vi "Get Size of Data from TD - Digital Data (Ramp 256 Samples) - Returns Correct Size.vi"() -> ()   [LabVIEW 2017, in "Composition.Tests.lvlib"]
uses:
  Composition.Tests.lvlib
  <vilib>/Waveform/DWDTOps.llb/Digital Pattern Generator (Ramp).vi
  <vilib>/addons/_JKI Toolkits/Caraya/classes/Assert/Assert Equal Value_Variant.vi
  Composition/Composition.lvlib
  <vilib>/addons/_JKI Toolkits/Caraya/classes/Assert/Assert.lvclass
  <vilib>/addons/_JKI Toolkits/Caraya/classes/Test/Test.lvclass
panel:
  out "error out":errorcluster
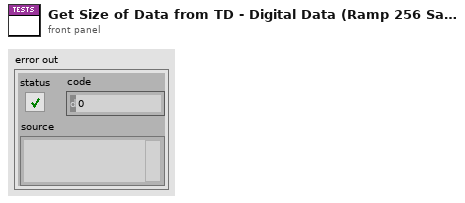
[diagram p1: front panel]
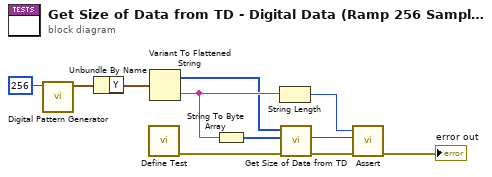
[diagram p0: block diagram]
diagram:
  n1 = call-poly <vilib>:"Digital Pattern Generator.vi"("number of samples"=u32 256) -> ("digital waveform"=w2:digitalwaveform)  [unwired: 9 in, 1 out]
  n2 = Unbundle By Name(w2) -> ("Y"=w1:digitaldata)
  n3 = call <vilib>:"Define Test.vi"() -> ("error out"=w7:errorcluster)  [unwired: 11 in]
  n4 = Variant To Flattened String(Variant=w1) -> (data string=w10:string, 1:w6:i16[])
  n5 = String To Byte Array(string=w10) -> (unsigned byte array=w4:u8[])
  n6 = String Length(string=w10) -> (length=w8:i32)
  n7 = call "Get Size of Data from TD.vi"("error in (no error)"=w7, "Data String"=w4, "Type Descriptor"=w6) -> ("error out"=w11:errorcluster, "Size of Data"=w5:i32)  [unwired: 7 in]
  n8 = call-poly <vilib>:"Assert.vi"("error in (no error)"=w11, "Y"=w5, "X"=w8) -> ("error out"=→"error out":errorcluster)  [unwired: 8 in]
